vi "Send Fuel.vi"(8 "error in":errorcluster, 11 "Fuel Flows":dbl[][](array[numeric])) -> (0 "error out":errorcluster)   [LabVIEW 2017, in "Akwizycja.lvlib"]
uses:
  Akwizycja.lvlib
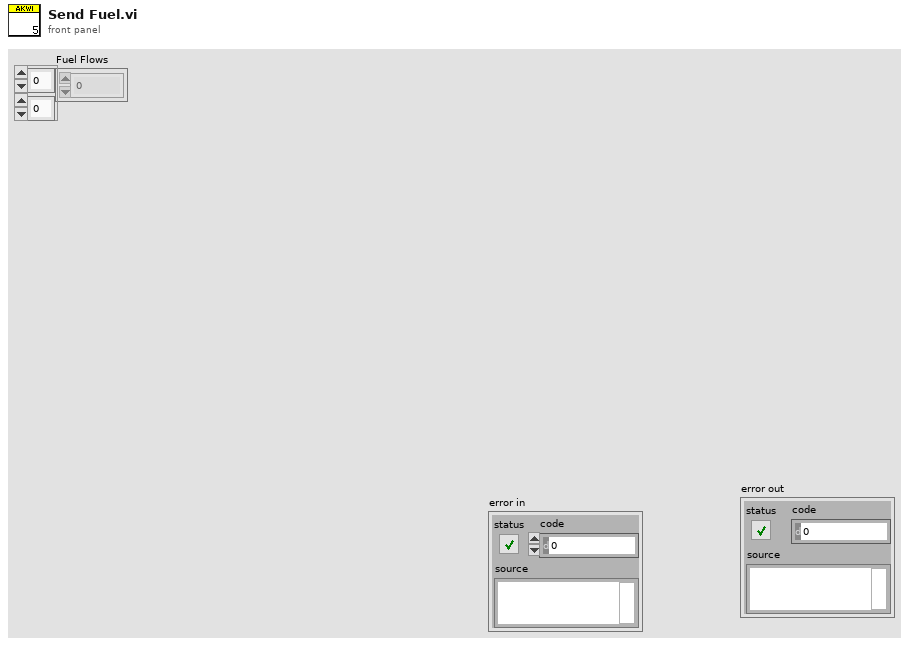
[diagram p1: front panel]
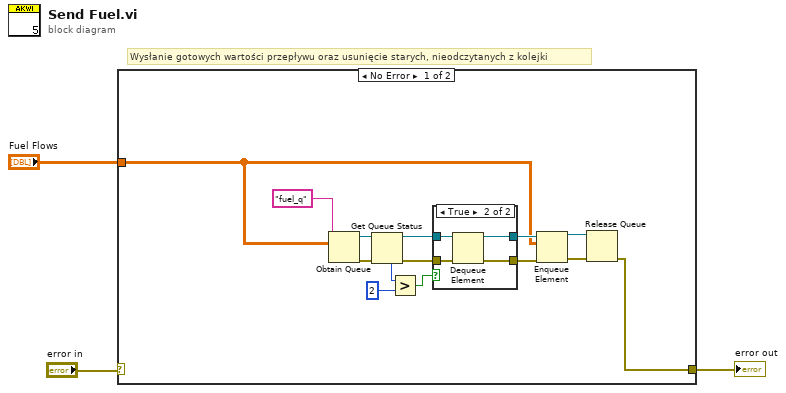
[diagram p0: block diagram]
diagram:
  # "Wysłanie gotowych wartości przepływu oraz usunięcie starych, nieodczytanych z kolejki"
  n1 = case shown="No Error" "error in" {
    selector: "error in" -> [_ w24]
    tunnel: [w4 w24] -> w2
    tunnel: "Fuel Flows" -> [w5 _]
    frame No Error {
      n2 = Obtain Queue(name (unnamed)="fuel_q", element data type=w5) -> (queue out=w7:refnum<queue>, error out=w6:errorcluster)  [unwired: 3 in, 1 out]
      n3 = Get Queue Status(queue=w7, error in (no error)=w6) -> (queue out=w11:refnum<queue>, error out=w13:errorcluster, # elements in queue=w12:i32)  [unwired: 1 in, 5 out]
      n4 = Greater?(x=w12, y=2) -> (0:w10:bool)
      n5 = case shown="True" w10 {
        tunnel: w13 -> [w18 w23]
        tunnel: w11 -> [w19 w22]
        tunnel: [w19 w21] -> w9
        tunnel: [w18 w20] -> w8
        frame False {
        }
        frame True {
          n6 = Dequeue Element(queue=w22, error in (no error)=w23) -> (queue out=w21:refnum<queue>, error out=w20:errorcluster)  [unwired: 1 in, 2 out]
        }
      }
      n7 = Enqueue Element(queue=w9, element=w5, error in (no error)=w8) -> (queue out=w15:refnum<queue>, error out=w14:errorcluster)  [unwired: 1 in, 1 out]
      n8 = Release Queue(queue=w15, error in (no error)=w14) -> (error out=w4:errorcluster)  [unwired: 1 in, 2 out]
    }
    frame Error {
    }
  }
  "error out" <- w2
